vi "Process movement controls.vi"(0 "Left":bool, 5 "Forward":bool, 7 "Right":bool, 9 "Speed":dbl, 11 "Direction":dbl) -> (6 "Speed":dbl, 10 "Direction":dbl)   [LabVIEW 2013]
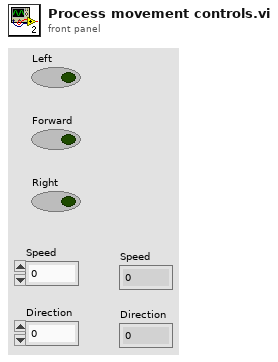
[diagram p1: front panel]
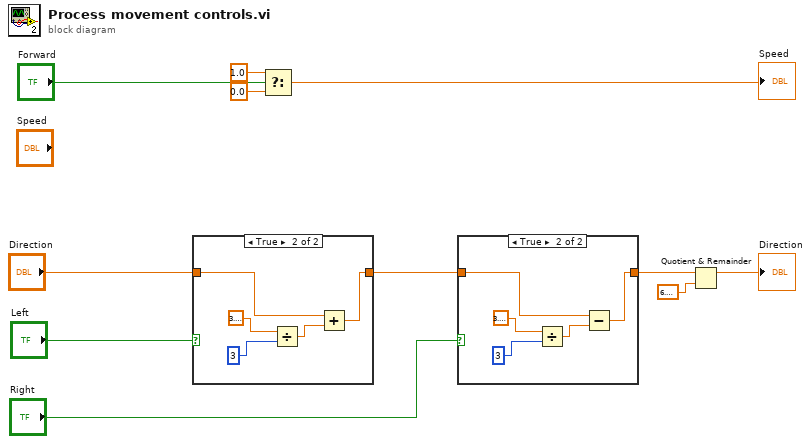
[diagram p0: block diagram]
diagram:
  n1 = case shown="True" "Left" {
    tunnel: "Direction" -> [w12 w14]
    tunnel: [w12 w13] -> w9
    frame False {
    }
    frame True {
      n2 = Divide(x=3.141592653589793, y=3) -> (x/y=w15:dbl)
      n3 = Add(x=w14, y=w15) -> (x+y=w13:dbl)
    }
  }
  n4 = Select(t=1.0, s="Forward", f=0.0) -> (s? t:f=→"Speed":dbl)
  n5 = case shown="True" "Right" {
    tunnel: w9 -> [w18 w20]
    tunnel: [w18 w19] -> w7
    frame False {
    }
    frame True {
      n6 = Divide(x=3.141592653589793, y=3) -> (x/y=w21:dbl)
      n7 = Subtract(x=w20, y=w21) -> (x-y=w19:dbl)
    }
  }
  n8 = Quotient & Remainder(x=w7, y=6.283185307179586) -> (x-y*floor(x/y)=→"Direction":dbl)  [unwired: 1 out]
